vi "PID is complete.vi"(6 "Error Threshold":dbl, 7 "sample length":i32=80, 8 "threshold":dbl=0.008, 9 "process variable":dbl, 10 "setpoint":dbl, 11 "PID Output":dbl) -> (2 "PID is Done?":bool, 3 "mean":dbl=0.00016497888749945157 format="%0.2f")   [LabVIEW 2018]
uses:
  <vilib>/ptbypt/NI_PtbyPt.lvlib
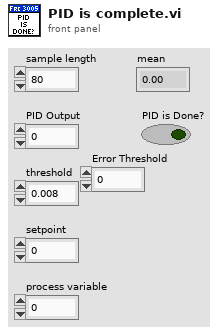
[diagram p1: front panel]
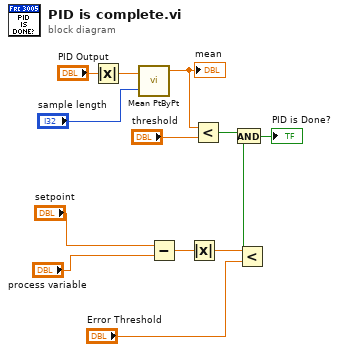
[diagram p0: block diagram]
diagram:
  n1 = Absolute Value(x="PID Output") -> (abs(x)=w7:dbl)
  n2 = call <vilib>:"Mean PtByPt.vi"("x"=w7, "sample length"="sample length") -> ("mean"=w9:dbl)  [unwired: 2 in, 1 out]
  "mean" <- w9
  n3 = Subtract(x="setpoint", y="process variable") -> (x-y=w4:dbl)
  n4 = Absolute Value(x=w4) -> (abs(x)=w3:dbl)
  n5 = Less?(x=w9, y="threshold") -> (x < y?=w8:bool)
  n6 = Less?(x=w3, y="Error Threshold") -> (x < y?=w2:bool)
  n7 = And(x=w8, y=w2) -> (x .and. y?=→"PID is Done?":bool)
